vi "DataBase - Initialize.vi"(8 "error in (no error)":errorcluster, 11 "VI In":refnum<vi>) -> (0 "error out":errorcluster, 3 "Event Registration Out":refnum<event-registration>)   [LabVIEW 2024, in "Data Base.lvlib"]
uses:
  Data Base.lvlib
  Support/General Type Defs/User Events Cluster.ctl
  DataBase Queue - Create.vi
  Support/User Events/User Events - Register Events.vi
  DataBase Queue - Enqueue.vi
  Support/User Events/User Events.lvlib
  Support/General Type Defs/General Type Defs.lvlib
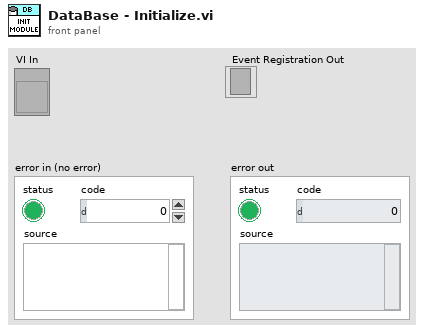
[diagram p1: front panel]
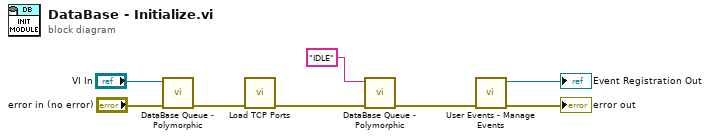
[diagram p0: block diagram]
diagram:
  n1 = call-poly "DataBase Queue - Polymorphic.vi"("error in"="error in (no error)", "VI In"="VI In") -> ("error out"=w2:errorcluster)  [unwired: 9 in]
  n2 = call "Load TCP Ports.vi"("error in"=w2) -> ("error out"=w1:errorcluster)  [unwired: 10 in]
  n3 = call-poly "DataBase Queue - Polymorphic.vi"("error in"=w1, "Message"="IDLE") -> ("error out"=w4:errorcluster)  [unwired: 9 in]
  n4 = call-poly "User Events - Manage Events.vi"("error in"=w4) -> ("error out"=→"error out":errorcluster, "Event Registration Out"=→"Event Registration Out":refnum<event-registration>)  [unwired: 9 in]
